vi "get #OfSegments.vi"(8 "error in (no error)":errorcluster caption="Fehler (Eingang, kein Fehler)", 11 "Test (Eingang)":refnum<class "Test.lvclass">) -> (0 "error out":errorcluster caption="Fehler (Ausgang)", 2 "#OfSegments":u32, 3 "Test (Ausgang)":refnum<class "Test.lvclass">)   [LabVIEW 2013, in "DatenKlassen.lvlib" / "Test.lvclass"]
uses:
  Test.lvclass
  Test.lvclass/Test.ctl
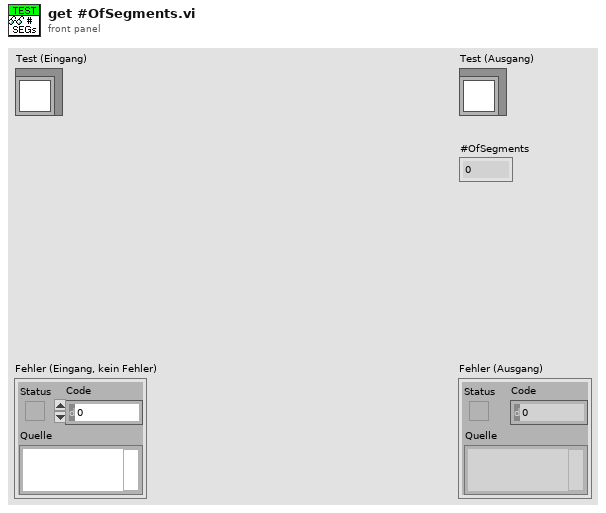
[diagram p1: front panel]
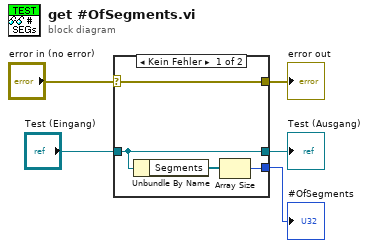
[diagram p0: block diagram]
diagram:
  n1 = case shown="Kein Fehler" "error in (no error)" {
    selector: "error in (no error)" -> [w9 w10]
    tunnel: [w9 w10] -> w4
    tunnel: [w8 w11] -> w2
    tunnel: "Test (Eingang)" -> [w8 w11]
    tunnel: [w6 _] -> w1
    frame No Error {
      n2 = Unbundle By Name(w8) -> ("Segments"=w7:refnum<class "Segment.lvclass">[])
      n3 = Array Size(array=w7) -> (size(s)=w6:i32)
    }
    frame Error {
    }
  }
  "error out" <- w4
  "Test (Ausgang)" <- w2
  "#OfSegments" <- w1
